vi "TestVirtual1.vi"(0 "reference in":refnum<class "IG#BaseInterface.lvclass">, 5 "error in (no error)":errorcluster) -> (14 "reference out":refnum<class "IG#BaseInterface.lvclass">, 15 "MethodName":string[](array[string]), 19 "error out":errorcluster)   [LabVIEW 2010, in "IG#BaseInterface.lvclass"]
uses:
  IG#BaseInterface.lvclass
  <vilib>/addons/_AddQ/G#Interface/G#Interface.lvclass
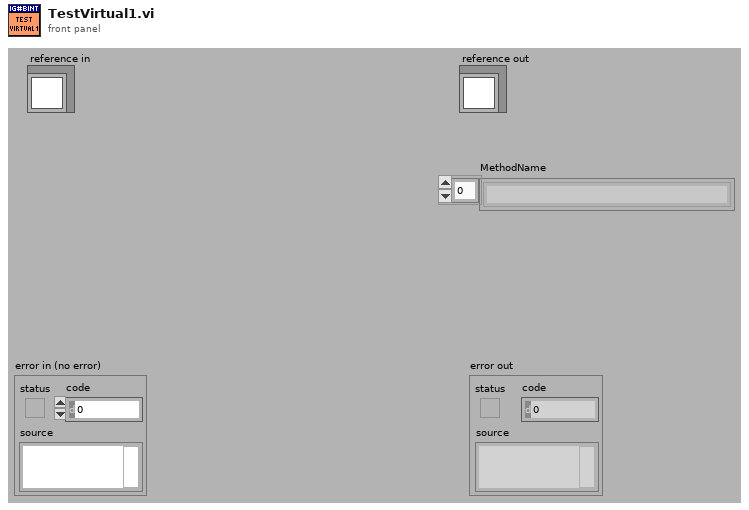
[diagram p1: front panel]
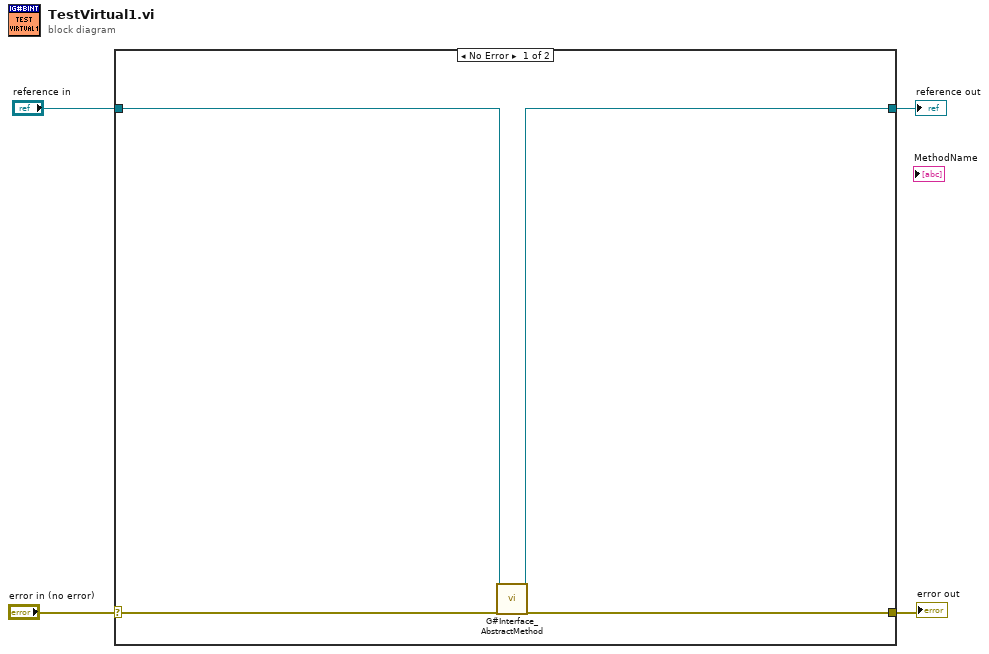
[diagram p0: block diagram]
diagram:
  n1 = case shown="No Error" "error in (no error)" {
    selector: "error in (no error)" -> [w7 w10]
    tunnel: [w8 w10] -> w3
    tunnel: [w5 w9] -> w1
    tunnel: "reference in" -> [w6 w9]
    frame No Error {
      n2 = call <vilib>:"G#Interface_AbstractMethod.vi"("reference in"=w6, "error in (no error)"=w7) -> ("reference out"=w5:refnum<class "IG#BaseInterface.lvclass">, "error out"=w8:errorcluster)  [unwired: 16 in]
    }
    frame Error {
    }
  }
  "error out" <- w3
  "reference out" <- w1
